vi "CreateSMOName.vi"(8 "error in (no error)":errorcluster) -> (0 "error out":errorcluster, 2 "Name":string)   [LabVIEW 2016, in "Instrument.Example.lvclass"]
uses:
  Instrument.Example.lvclass
  <userlib>/LevyLab/Levylab Instruments/SMOs/Instrument/Instrument.lvclass
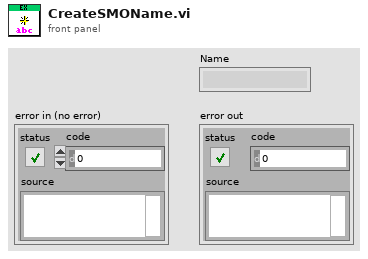
[diagram p1: front panel]
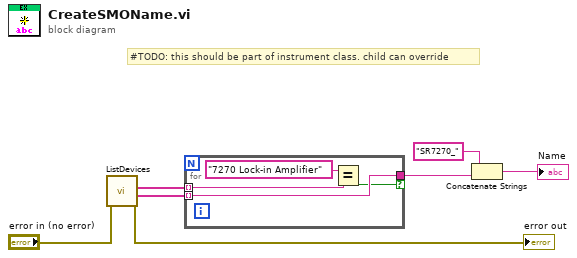
[diagram p0: block diagram]
diagram:
  # "#TODO: this should be part of instrument class. child can override"
  n1 = call <userlib>:"ListDevices.vi"("error in (no error)"="error in (no error)") -> ("error out"=→"error out":errorcluster, "Serial Numbers"=w4:string[], "Product Names"=w3:string[])  [unwired: 7 in, 1 out]
  n2 = for {
    tunnel: w3 -> [w10] mode=indexing
    tunnel: w4 -> [w9] mode=indexing
    tunnel: [w9] -> w6 if=w8
    n3 = Equal?(x="7270 Lock-in Amplifier", y=w10) -> (x = y?=w8:bool)
  }
  n4 = Concatenate Strings("SR7270_", w6) -> (→"Name":string)
